vi "Condition Name.vi"(6 "Terminals (All Msg Output)":T1, 8 "error in":errorcluster, 9 "Terminals (All Msg Input)":T1, 10 "Name":T2) -> (0 "error out":errorcluster)   [LabVIEW 2020, in "_Rescript.lvlib" / "Msg.lvlib" / "Msg.lvclass"]
uses:
  Msg.lvclass
  _Rescript.lvlib
  Name.ctl
  Terminals.ctl
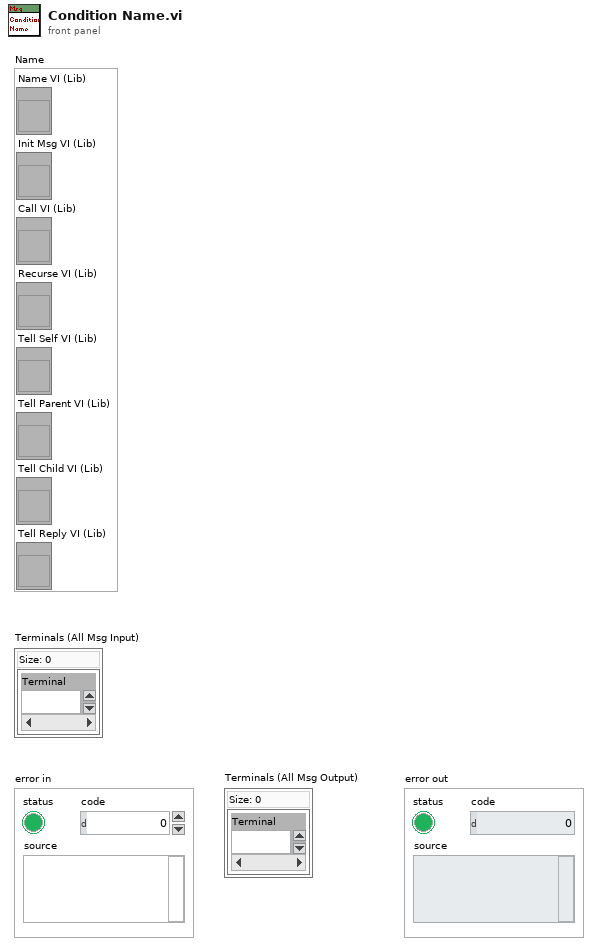
[diagram p1: front panel]
types:
  T1 = typedef "_Rescript.lvlib/Terminals.ctl" = set{i32}
  T2 = typedef "_Rescript.lvlib/Msg.lvlib/Msg.lvclass/Name.ctl" = cluster{"Name VI (Lib)":refnum<vi>, "Init Msg VI (Lib)":refnum<vi>, "Call VI (Lib)":refnum<vi>, "Recurse VI (Lib)":refnum<vi>, "Tell Self VI (Lib)":refnum<vi>, "Tell Parent VI (Lib)":refnum<vi>, "Tell Child VI (Lib)":refnum<vi>, "Tell Reply VI (Lib)":refnum<vi>}
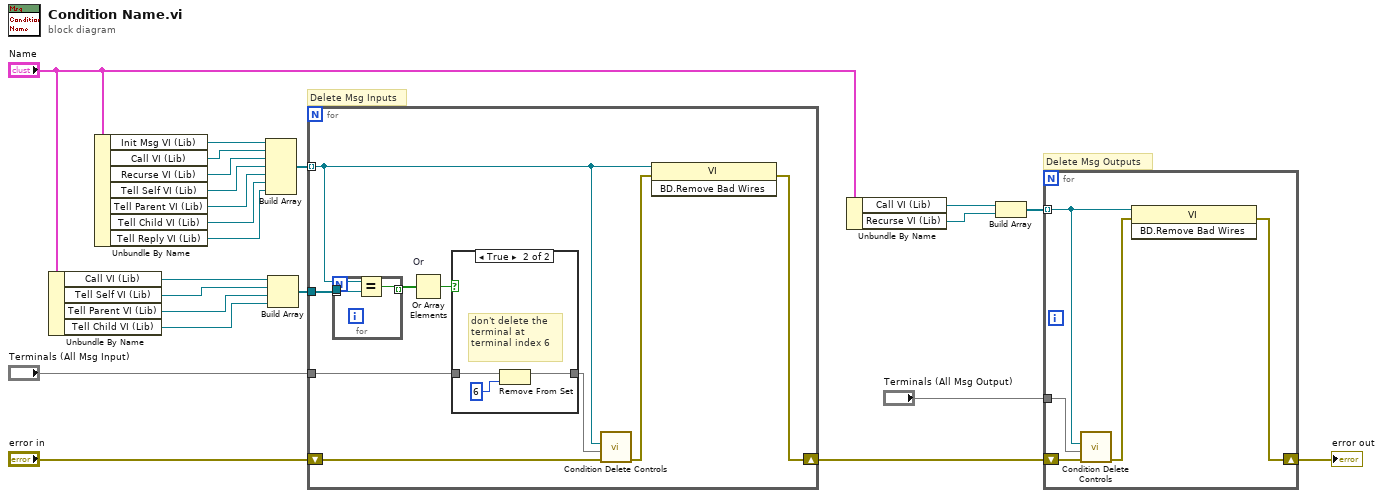
[diagram p0: block diagram]
diagram:
  # "Delete Msg Outputs"
  # "Delete Msg Inputs"
  n1 = Unbundle By Name("Name") -> ("Call VI (Lib)"=w5:refnum<vi>, "Tell Self VI (Lib)"=w4:refnum<vi>, "Tell Parent VI (Lib)"=w3:refnum<vi>, "Tell Child VI (Lib)"=w2:refnum<vi>)
  n2 = Unbundle By Name("Name") -> ("Init Msg VI (Lib)"=w17:refnum<vi>, "Call VI (Lib)"=w6:refnum<vi>, "Recurse VI (Lib)"=w14:refnum<vi>, "Tell Self VI (Lib)"=w7:refnum<vi>, "Tell Parent VI (Lib)"=w8:refnum<vi>, "Tell Child VI (Lib)"=w11:refnum<vi>, "Tell Reply VI (Lib)"=w15:refnum<vi>)
  n3 = Build Array(w17, w6, w14, w7, w8, w11, w15) -> (w16:refnum<vi>[])
  n4 = Build Array(w5, w4, w3, w2) -> (w10:refnum<vi>[])
  n5 = for {
    tunnel: "Terminals (All Msg Input)" -> [w28]
    shift-right: [w29] -> w21
    shift-left: "error in" -> [w31]
    tunnel: w16 -> [w25] mode=indexing
    tunnel: w10 -> [w26]
    n6 = for {
      tunnel: w26 -> [w37] mode=indexing
      tunnel: w25 -> [w38]
      tunnel: [w36] -> w24 mode=indexing
      n7 = Equal?(x=w38, y=w37) -> (x = y?=w36:bool)
    }
    n8 = Or Array Elements "Or"(Boolean array=w24) -> (logical OR=w23:bool)
    n9 = case shown="True" w23 {
      tunnel: w28 -> [w32 w34]
      tunnel: [w32 w33] -> w27
      frame False {
      }
      frame True {
        # "don't delete the terminal at terminal index 6"
        n10 = Remove From Set(10:6 ("Numeric"), 11:w34) -> (3:w33:T1)  [unwired: 1 out]
      }
    }
    n11 = call "Condition Delete Controls.vi"("error in"=w31, "Terminals"=w27, "VI"=w25) -> ("error out"=w30:errorcluster)  [unwired: 8 in]
    n12 = invoke class="VI" method="BD.Remove Bad Wires"(reference=w25, error in=w30) -> (error out=w29:errorcluster)  [unwired: 1 in, 2 out]
  }
  n13 = Unbundle By Name("Name") -> ("Call VI (Lib)"=w9:refnum<vi>, "Recurse VI (Lib)"=w19:refnum<vi>)
  n14 = Build Array(w9, w19) -> (w18:refnum<vi>[])
  n15 = for {
    tunnel: "Terminals (All Msg Output)" -> [w39]
    shift-right: [w41] -> w20
    shift-left: w21 -> [w43]
    tunnel: w18 -> [w40] mode=indexing
    n16 = call "Condition Delete Controls.vi"("error in"=w43, "Terminals"=w39, "VI"=w40) -> ("error out"=w42:errorcluster)  [unwired: 8 in]
    n17 = invoke class="VI" method="BD.Remove Bad Wires"(reference=w40, error in=w42) -> (error out=w41:errorcluster)  [unwired: 1 in, 2 out]
  }
  "error out" <- w20
